vi "DMC_Open.vi"(6 "Invert (F)":bool, 7 "encoderTicks":i32, 8 "error in (no error)":errorcluster, 9 "gearRatio":i32, 10 "wheelDiametermm":dbl, 11 "Device Number":u8) -> (0 "error out":errorcluster, 3 "output cluster":T1={"DeviceStatus"={"status"=FALSE, "code"=0, "source"=""}, "Type"=enum."PWM", "PWM"={"PWM Channel"=enum."Invalid", "DeadBand"={"Name"="", "maxPositivePwm"=0, "minPositivePwm"=0, "centerPwm"=0, "maxNegativePwm"=0, "minNegativePwm"=0, "angularRange"=0}}, "CAN"={"Device Number"=0, "SetOutput VI Ref"=variant, "GetOutput VI Ref"=variant, "Enable VI Ref"=variant, "Disable VI Ref"=variant, "Data"=variant}, "Invert"=FALSE, "DIO PWM"={"PWM \"Enable\" Channel"=enum."Invalid", "DIOChannel"=enum."Invalid", "PWM Rate"=0.0}})   [LabVIEW 2018, in "DMC60C.lvlib"]
uses:
  <vilib>/Rock Robotics/WPI/ThirdParty/TopLevel/DMC60C/DMC60C.lvlib
  <vilib>/Rock Robotics/WPI/MotorControl/WPI_MotorControlDeviceRef.ctl
  <vilib>/Rock Robotics/WPI/MotorControl/WPI_MotorControlType.ctl
  <vilib>/Rock Robotics/SystemInterfaces/DIO/FPGA_DIOPWMChannel.ctl
  <vilib>/Rock Robotics/WPI/PWM/WPI_PWMDeadband.ctl
  <vilib>/Rock Robotics/SystemInterfaces/DIO/FPGA_DIOChannel.ctl
  <vilib>/Rock Robotics/WPI/ThirdParty/TopLevel/DMC60C/DMC60CDeviceRef.ctl
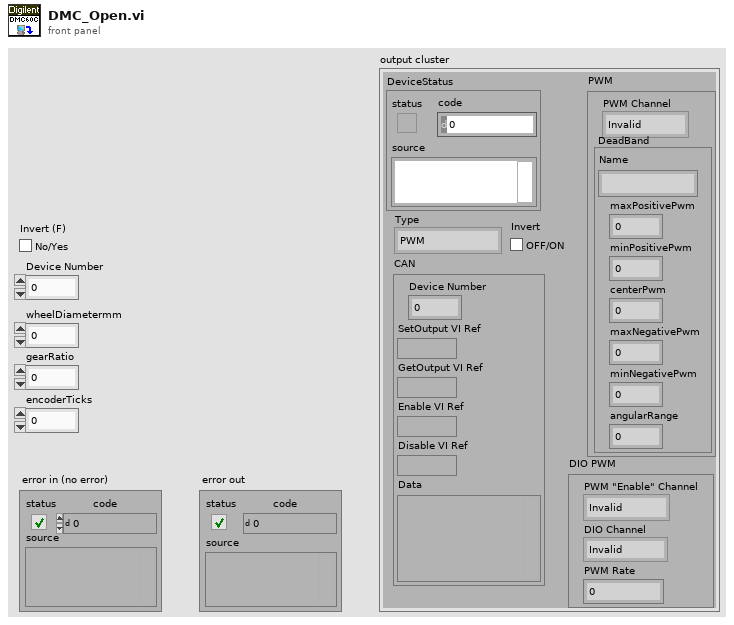
[diagram p1: front panel]
types:
  T1 = typedef "WPI_MotorControlDeviceRef.ctl" = cluster{"DeviceStatus":errorcluster, "Type":T2, "PWM":cluster{"PWM Channel":T3, "DeadBand":T4}, "CAN":cluster{"Device Number":u8, "SetOutput VI Ref":variant, "GetOutput VI Ref":variant, "Enable VI Ref":variant, "Disable VI Ref":variant, "Data":variant}, "Invert":bool, "DIO PWM":cluster{"PWM \"Enable\" Channel":T3, "DIOChannel":T5, "PWM Rate":dbl}}
  T2 = typedef "WPI_MotorControlType.ctl" = enum16{"PWM", "CAN", "DIO PWM"}
  T3 = typedef "FPGA_DIOPWMChannel.ctl" = enum8{"PWM 0", "PWM 1", "PWM 2", "PWM 3", "PWM 4", "PWM 5", "PWM 6", "PWM 7", "PWM 8", "PWM 9", "PWM MXP 0", "PWM MXP 1", "PWM MXP 2", "PWM MXP 3", "PWM MXP 4", "PWM MXP 5", "PWM MXP 6", "PWM MXP 7", "PWM MXP 8", "PWM MXP 9", "Invalid"}
  T4 = typedef "WPI_PWMDeadband.ctl" = cluster{"Name":string, "maxPositivePwm":i32, "minPositivePwm":i32, "centerPwm":i32, "maxNegativePwm":i32, "minNegativePwm":i32, "angularRange":u16}
  T5 = typedef "FPGA_DIOChannel.ctl" = enum8{"DIO 0", "DIO 1", "DIO 2", "DIO 3", "DIO 4", "DIO 5", "DIO 6", "DIO 7", "DIO 8", "DIO 9", "DIO MXP 0", "DIO MXP 1", "DIO MXP 2", "DIO MXP 3", "DIO MXP 4", "DIO MXP 5", "DIO MXP 6", "DIO MXP 7", "DIO MXP 8", "DIO MXP 9", "DIO MXP 10", "DIO MXP 11", "DIO MXP 12", "DIO MXP 13", "DIO MXP 14", "DIO MXP 15", "SPI Port CS1", "SPI Port CS2", "SPI Port CS3", "SPI Port MISO", "SPI Port MOSI", "Invalid"}
  T6 = typedef "DMC60C.lvlib/DMC60CDeviceRef.ctl" = cluster{"DeviceRef":i32, "arbID":u32}
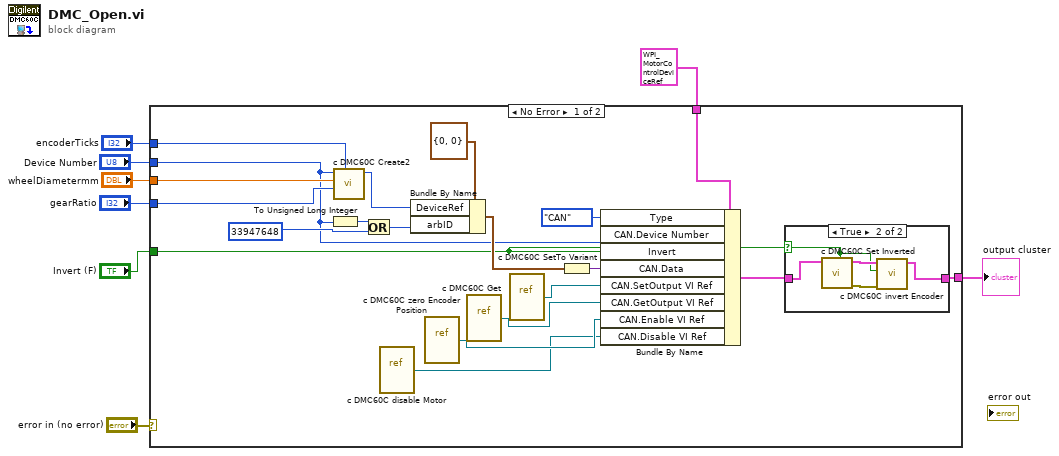
[diagram p0: block diagram]
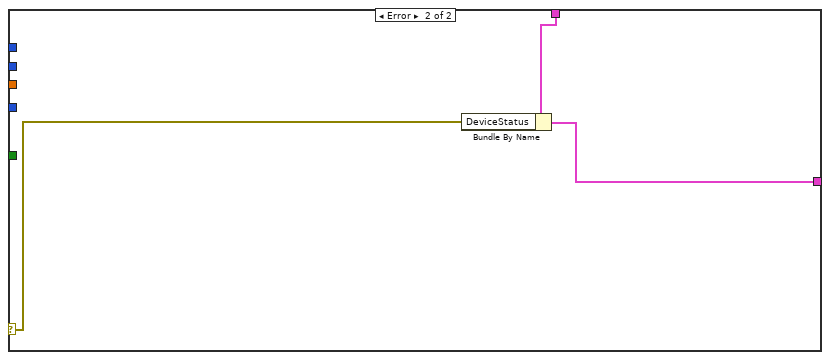
[diagram p3: hidden frame]
diagram:
  n1 = case shown="No Error" "error in (no error)" {
    selector: "error in (no error)" -> [_ w36]
    tunnel: "Device Number" -> [w12 _]
    tunnel: "wheelDiametermm" -> [w28 _]
    tunnel: "gearRatio" -> [w27 _]
    tunnel: "encoderTicks" -> [w26 _]
    tunnel: T1 {"DeviceStatus"={"status"=FALSE, "code"=0, "source"=""}, "Type"=enum."PWM", "PWM"={"PWM Channel"=enum."Invalid", "DeadBand"={"Name"="", "maxPositivePwm"=0, "minPositivePwm"=0, "centerPwm"=0, "maxNegativePwm"=0, "minNegativePwm"=0, "angularRange"=0}}, "CAN"={"Device Number"=0, "SetOutput VI Ref"=variant, "GetOutput VI Ref"=variant, "Enable VI Ref"=variant, "Disable VI Ref"=variant, "Data"=variant}, "Invert"=FALSE, "DIO PWM"={"PWM \"Enable\" Channel"=enum."Invalid", "DIOChannel"=enum."Invalid", "PWM Rate"=0.0}} ("MotorControlDeviceRef") -> [w23 w37]
    tunnel: "Invert (F)" -> [w11 _]
    tunnel: [w9 w35] -> w1
    frame No Error {
      n2 = To Unsigned Long Integer(number=w12) -> (unsigned 32bit integer=w19:u32)
      n3 = call <vilib>:"c DMC60C Create2.vi"("encoderTicks"=w26, "gearRatio"=w27, "wheelDiametermm"=w28, "deviceNumber"=w12) -> ("function return"=w24:i32)  [unwired: 6 in, 1 out]
      n4 = Or(x=w19, y=u32 33947648) -> (x .or. y?=w21:u32)
      n5 = vi-ref <vilib>:"c DMC60C disable Motor.vi"() -> (w13:refnum<vi>)
      n6 = Bundle By Name(cluster=T6 {"DeviceRef"=0, "arbID"=0}, "DeviceRef"=w24, "arbID"=w21) -> (w17:T6)
      n7 = vi-ref <vilib>:"c DMC60C zero Encoder Position.vi"() -> (w14:refnum<vi>)
      n8 = vi-ref <vilib>:"c DMC60C Get.vi"() -> (w15:refnum<vi>)
      n9 = vi-ref <vilib>:"c DMC60C Set.vi"() -> (w16:refnum<vi>)
      n10 = To Variant(anything=w17) -> (Variant=w18:variant)
      n11 = Bundle By Name(cluster=w23, "Type"=WPI_MotorControlType."CAN", "CAN.Device Number"=w12, "Invert"=w11, "CAN.Data"=w18, "CAN.SetOutput VI Ref"=w16, "CAN.GetOutput VI Ref"=w15, "CAN.Enable VI Ref"=w14, "CAN.Disable VI Ref"=w13) -> (w10:T1)
      n12 = case shown="True" w11 {
        selector: w11 -> [_ w31]
        tunnel: w10 -> [w29 w34]
        tunnel: [w29 w30] -> w9
        frame False {
        }
        frame True {
          n13 = call <vilib>:"c DMC60C Set Inverted.vi"("isInverted"=w31, "DMC60DevRef"=w34) -> ("error out"=w33:errorcluster, "DMC60DevRef"=w32:T1)  [unwired: 8 in]
          n14 = call <vilib>:"c DMC60C invert Encoder.vi"("error in (no error)"=w33, "isInverted"=w31, "DMC60DevRef"=w32) -> ("DMC60DevRef"=w30:T1)  [unwired: 7 in, 1 out]
        }
      }
    }
    frame Error {
      n15 = Bundle By Name(cluster=w37, "DeviceStatus"=w36) -> (w35:T1)
    }
  }
  "output cluster" <- w1
